vi "Check open batches .vi"(7 "error in (no error) 5":errorcluster, 10 "Module Number  2":dbl=1.0) -> (0 "error out":errorcluster, 3 "Open New Batch":bool)   [LabVIEW 2015, in "Copy of Untitled Library 1.lvlib"]
uses:
  Copy of Untitled Library 1.lvlib
  Controls/Enum Constant.ctl
  <userlib>/origin_lib_main/db_interface/DB Operations Enum.ctl
  <userlib>/origin_lib_main/ui_msg_lib/CTRL/Display MSG Types.ctl
  <vilib>/addons/database/_DB Variant To Data/Database Variant To Data.xnode
  <userlib>/origin_lib_main/db_interface/DB Interface.lvlib
  <userlib>/origin_lib_main/ui_msg_lib/MSG Library.lvlib
panel:
  in  "error in (no error) 6":errorcluster
  out "format string 2":string
  out "Open Batch or Not?":bool
  out "subarray":string[](array[string])
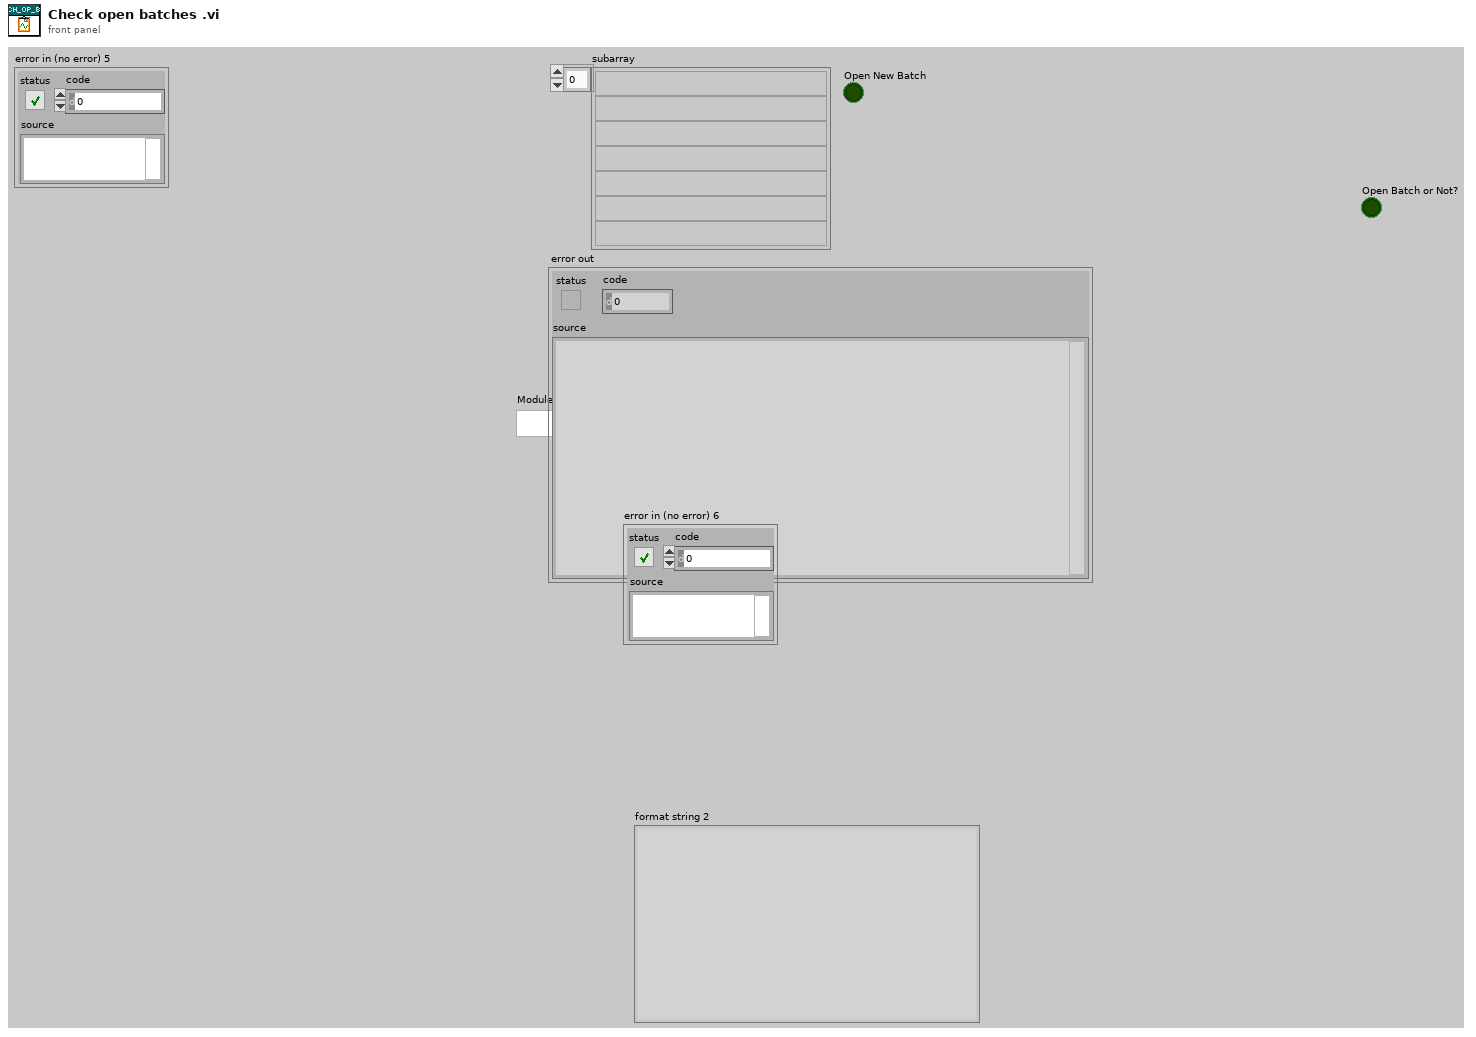
[diagram p1: front panel]
types:
  T1 = typedef "DB Interface.lvlib/DB Operations Enum.ctl" = enum16{"Select", "Update", "Insert", "Delete", "Fetch SQL Query", "Execute SQL Query", "Drop Table", "List Tables"}
  T2 = typedef "Enum Constant.ctl" = enum16{"Init", "Read", "Write"}
  T3 = typedef "FGV Data.ctl" = T4[]
  T4 = typedef "FGV Cluster Data.ctl" = cluster{"Manual/Automatic":bool, "UI Controllers ":string[], "UI Primery Key ":dbl[], "Caller Queue & MSG":T5, "Module ID":dbl, "DB Reference In":T6, "Products Columns":string[], "Cluster":cluster{"Delete Product":enum8{"Enabled", "Disabled", "Disabled and Grayed Out"}, "Add Product ":enum8{"Enabled", "Disabled", "Disabled and Grayed Out"}, "EDIT BATCH":enum8{"Enabled", "Disabled", "Disabled and Grayed Out"}, "Open Batch ":enum8{"Enabled", "Disabled", "Disabled and Grayed Out"}, "Close Batch":enum8{"Enabled", "Disabled", "Disabled and Grayed Out"}, "Delete Batch":enum8{"Enabled", "Disabled", "Disabled and Grayed Out"}, "Add Batch ":enum8{"Enabled", "Disabled", "Disabled and Grayed Out"}}}
  T5 = typedef "Queue and Caller MSG.ctl" = cluster{"Caller Queue":refnum<queue>, "Caller MSG":string}
  T6 = typedef "NI_Database_API.lvlib/Conn ObjectReference.ctl" = refnum<k1>
  T7 = typedef "MSG Library.lvlib/Display MSG Types.ctl" = enum16{"Display MSG 1", "Display MSG 2", "Display MSG Load", "End MSG Load ", "Display 2 STR MSG"}
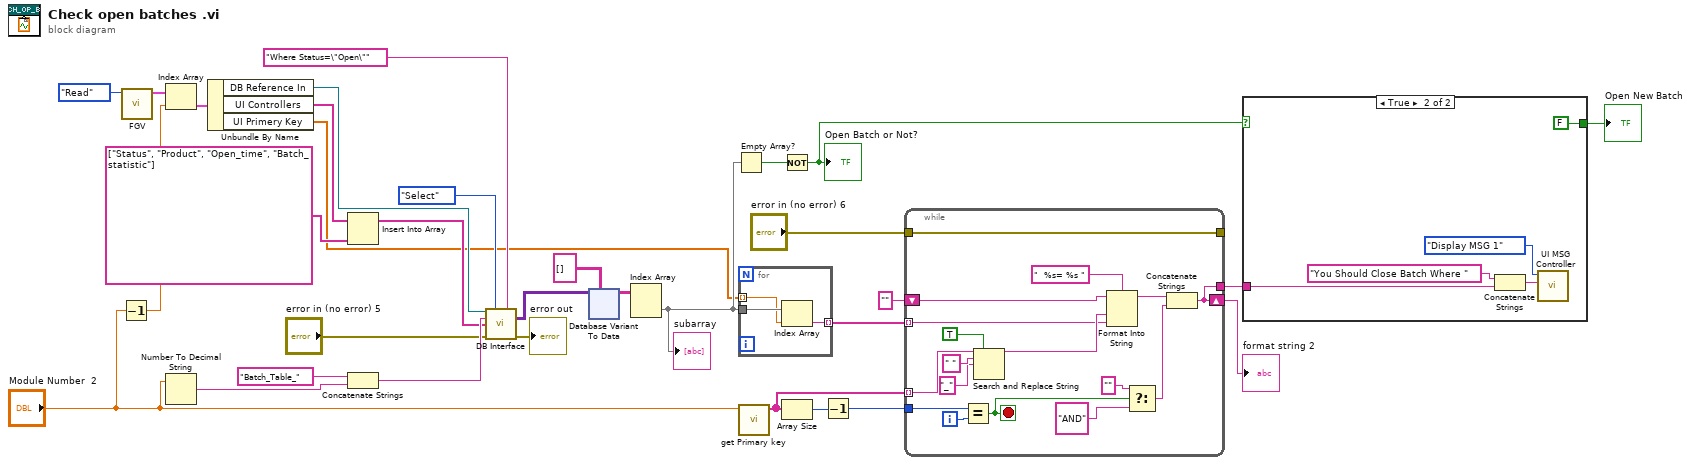
[diagram p0: block diagram]
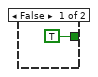
[diagram p2: hidden frame]
diagram:
  n1 = Decrement(x="Module Number  2") -> (x-1=w25:dbl)
  n2 = call "FGV.vi"("Enum"=Enum_Constant."Read") -> ("Read Data"=w27:T3)  [unwired: 9 in, 1 out]
  n3 = Index Array(array=w27, index=w25) -> (element=w26:T4)
  n4 = Number To Decimal String(number="Module Number  2") -> (decimal integer string=w29:string)  [unwired: 1 in]
  n5 = Unbundle By Name(w26) -> ("DB Reference In"=w20:T6, "UI Controllers"=w19:string[], "UI Primery Key"=w11:dbl[])
  n6 = Insert Into Array(array=w19, new element=string[] ["Status", "Product", "Open_time", "Batch_statistic"] ("element")) -> (w16:string[])  [unwired: 1 in]
  n7 = Concatenate Strings("Batch_Table_" ("string"), w29) -> (w28:string)
  n8 = call <userlib>:"DB Interface.vi"("DB Ref In"=w20, "Operation"=DB_Operations_Enum."Select", "condition"="Where Status=\"Open\"", "DB Table"=w28, "DB columns"=w16, "error in (no error)"="error in (no error) 5") -> ("data Out"=w22:variant[][], "error out"=→"error out":errorcluster)  [unwired: 6 in, 2 out]
  n9 = xnode "Database Variant To Data"("database variant"=w22, "type"=string[][] [] ("columns")) -> ("data"=w23:string[][])  [unwired: 1 in, 1 out]
  n10 = Index Array(array=w23) -> (element=w12:string[])  [unwired: 2 in]
  "subarray" <- w12
  n11 = Empty Array?(array=w12) -> (empty?=w14:bool)
  n12 = for {
    tunnel: w12 -> [w35]
    tunnel: w11 -> [w34] mode=indexing
    tunnel: [w33] -> w4 mode=indexing
    n13 = Index Array(array=w35, index=w34) -> (element=w33:string)
  }
  n14 = call "get Primary key.vi"("Module Number"="Module Number  2") -> ("Primery Key"=w5:string[])  [unwired: 10 in]
  n15 = Not(x=w14) -> (.not. x?=w13:bool)
  "Open Batch or Not?" <- w13
  n16 = Array Size(array=w5) -> (size(s)=w9:i32)
  n17 = Decrement(x=w9) -> (x-1=w8:i32)
  n18 = while {
    shift-right: [w36] -> w7
    shift-left: "" ("format string") -> [w51]
    tunnel: w8 -> [w45]
    tunnel: [w39] -> _
    tunnel: "error in (no error) 6" -> [w39]
    tunnel: w5 -> [w38] mode=indexing
    tunnel: w4 -> [w37] mode=indexing
    tunnel: [w36] -> w3
    i -> [w46]
    stop <- w40 stop-if-true
    n19 = Equal?(x=w45, y=w46) -> (x = y?=w40:bool)
    n20 = Search and Replace String(replace all?=TRUE ("replace all? (F)"), input string=w38, search string=" ", replace string="_" ("replace string (\"\")")) -> (result string=w41:string)  [unwired: 4 in, 3 out]
    n21 = Format Into String(format string="  %s= %s ", initial string=w51, w41, w37) -> (resulting string=w50:string)  [unwired: 1 in, 1 out]
    n22 = Select(t="", s=w40, f="AND") -> (s? t:f=w47:string)
    n23 = Concatenate Strings(w50, w47) -> (w36:string)
  }
  "format string 2" <- w7
  n24 = case shown="True" w13 {
    tunnel: [TRUE FALSE] -> w1
    tunnel: w3 -> [_ w55]
    frame False {
    }
    frame True {
      n25 = Concatenate Strings("You Should Close Batch Where " ("string"), w55) -> (w54:string)
      n26 = call <userlib>:"UI MSG Controller.vi"("MSG"=w54, "Display MSG Type"=Display_MSG_Types."Display MSG 1") -> ()  [unwired: 6 in, 4 out]
    }
  }
  "Open New Batch" <- w1
